vi "类型1自动误差计算.vi"(8 "允许误差":dbl, 9 "模拟量量程范围":dbl, 10 "设定值_1":dbl, 11 "反馈值_1":dbl format="%.6f") -> (1 "字符串_误差_1":string, 2 "误差_1":dbl, 3 "合格_1?":bool)   [LabVIEW 2010]
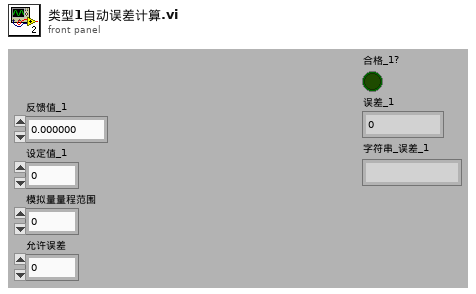
[diagram p1: front panel]
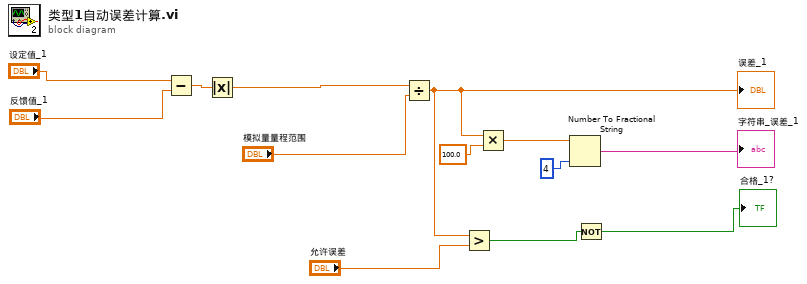
[diagram p0: block diagram]
diagram:
  n1 = Subtract(x="设定值_1", y="反馈值_1") -> (x-y=w13:dbl)
  n2 = Absolute Value(x=w13) -> (abs(x)=w11:dbl)
  n3 = Divide(x=w11, y="模拟量量程范围") -> (x/y=w1:dbl)
  "误差_1" <- w1
  n4 = Greater?(x=w1, y="允许误差") -> (0:w4:bool)
  n5 = Multiply(x=w1, y=100.0) -> (x*y=w2:dbl)
  n6 = Number To Fractional String(number=w2, precision (6)=i16 4 ("精度(6)")) -> (F-format string=→"字符串_误差_1":string)  [unwired: 2 in]
  n7 = Not(x=w4) -> (.not. x?=→"合格_1?":bool)
